vi "Close Motor Communication.vi"   [LabVIEW 2017, in "NI_Robotics_Motor Communication.lvclass"]
doc: "Terminates a communication session between a motor and the wheel the motor controls. Wire data to the <B>motor communication in</B> input to determine the polymorphic instance to use or manually select the instance."
uses:
  <vilib>/robotics/Actuation/Motor Communication/NI_Robotics_Motor Communication.lvclass
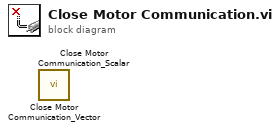
[diagram p0: block diagram]
diagram:
  n1 = call <vilib>:"Close Motor Communication_Vector.vi"() -> ()  [unwired: 11 in, 1 out]
  n2 = call <vilib>:"Close Motor Communication_Scalar.vi"() -> ()  [unwired: 11 in, 1 out]
